vi "Jenkins - Get Job Number.vi"(8 "error in (no error)":errorcluster, 10 "Script Job Name (Within Build Script Folder)":string, 11 "IP Address":string) -> (0 "error out":errorcluster, 3 "Job Number":i32)   [LabVIEW 2014]
uses:
  <vilib>/Utility/error.llb/Error Cluster From Error Code.vi
  <vilib>/ErrorRing/Error Ring.xnode
  <vilib>/httpClient/LabVIEWHTTPClient.lvlib
  <vilib>/wsapi/NI_WebServices.lvlib
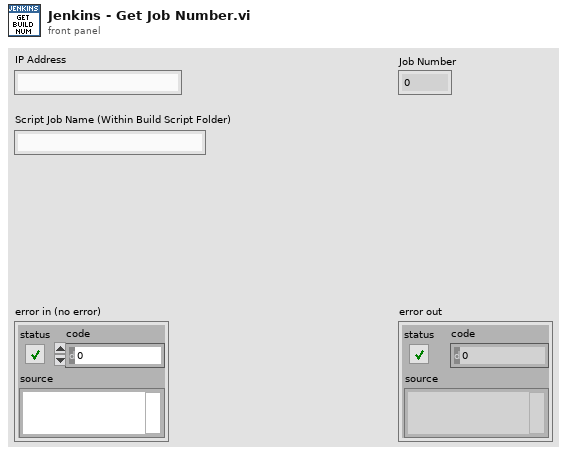
[diagram p1: front panel]
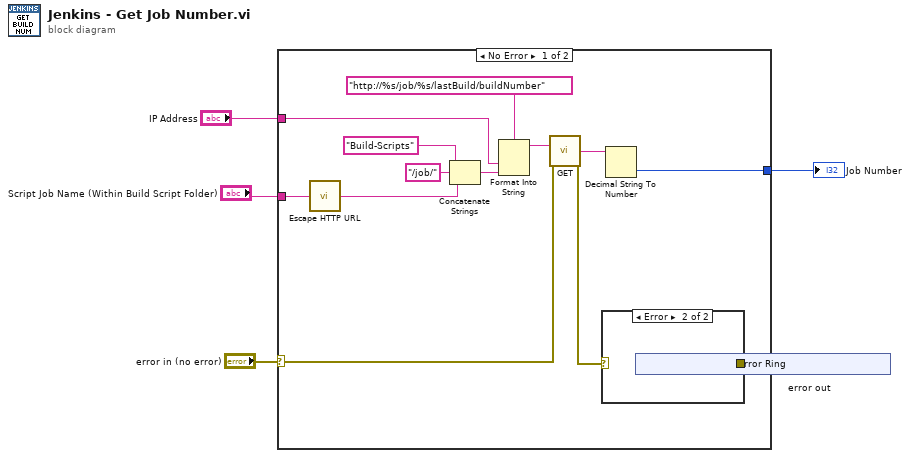
[diagram p0: block diagram]
diagram:
  n1 = case shown="No Error" "error in (no error)" {
    selector: "error in (no error)" -> [w8 w26]
    tunnel: "IP Address" -> [w12 _]
    tunnel: [w6 w26] -> w4
    tunnel: [w11 _] -> w3
    tunnel: "Script Job Name (Within Build Script Folder)" -> [w10 _]
    frame No Error {
      n2 = call <vilib>:"Escape HTTP URL.vi"("unescaped string in"=w10) -> ("escaped string out"=w9:string)
      n3 = Concatenate Strings("Build-Scripts" ("JSON"), "/job/" ("string"), w9) -> (w13:string)
      n4 = Format Into String(format string="http://%s/job/%s/lastBuild/buildNumber", w12, w13) -> (resulting string=w18:string)  [unwired: 2 in, 1 out]
      n5 = call <vilib>:"GET.vi"("url"=w18, "error in (no error)"=w8) -> ("body"=w14:string, "error out"=w7:errorcluster)  [unwired: 10 in, 2 out]
      n6 = case shown="Error" w7 {
        selector: w7 -> [w19 _]
        tunnel: [w19 w20] -> w6
        frame No Error {
        }
        frame Error {
          n7 = xnode "Error Ring"() -> ("error out"=w20:errorcluster)
        }
      }
      n8 = Decimal String To Number(string=w14) -> (number=w11:i32)  [unwired: 2 in, 1 out]
    }
    frame Error {
    }
  }
  "error out" <- w4
  "Job Number" <- w3
